vi "test_read-nmea-data2.vi"() -> ()   [LabVIEW 2019]
uses:
  <vilib>/Utility/file.llb/Write Delimited Spreadsheet (string).vi
panel:
  out "Array 2":string[](array[string])
  out "Numeric":i32=9674
  out "Array":string[](array[string])
  out "before substring":string
  in  "text":string="15:08:57.26\tF9P\t$GNRMC,060859.00,A,3723.60792,N,12656.91690,E,0.042,,250720,,,A,V*1C\n\t\n15:08:57.28\tF9P\t$GNVTG,,T,,M,0.042,N,0.078,K,A*34\n\t\n15:08:57.30\tF9P\t$GNGGA,060859.00,3723.60792,N,12656.91690,E,1,12,0.63,59.1,M,18.5,M,,*79\n\t\n15:08:57.32\tF9P\t$GNGSA,A,3,12,06,19,05,17,09,04,02,,,,,1.16,0.63,0.97,1*0D\n\t\n15:08:57.34\tF9P\t$GNGSA,A,3,70,85,71,84,,,,,,,,,1.16,0.63,0.97,2*0F\n\t\n15:08:57.36\tF9P\t$GNGSA,A,3,36,19,11,04,09,12,,,,,,,1.16,0.63,0.97,3*0D\n\t\n15:08:57.38\tF9P\t$GNGSA,A,3,14,11,33,,,,,,,,,,1.16,0.63,0.97,4*0C\n\t\n15:08:57.40\tF9P\t$GPGSV,3,1,09,02,53,317,32,04,19,045,33,05,36,246,36,06,65,044,35,1*64\n\t\n15:08:57.42\tF9P\t$GPGSV,3,2,09,09,45,076,33,12,24,278,37,17,35,153,31,19,54,156,27,1*62\n\t\n15:08:57.44\tF9P\t$GPGSV,3,3,09,25,12,308,17,1*54\n\t\n15:08:57.46\tF9P\t$GPGSV,3,1,09,02,53,317,,04,19,045,25,05,36,246,25,06,65,044,23,6*60\n\t\n15:08:57.48\tF9P\t$GPGSV,3,2,09,09,45,076,27,12,24,278,13,17,35,153,14,19,54,156,,6*64\n\t\n15:08:57.50\tF9P\t$GPGSV,3,3,09,25,12,308,,6*55\n\t\n15:08:57.52\tF9P\t$GLGSV,2,1,08,69,13,031,,70,73,042,31,71,50,204,30,72,03,209,,1*70\n\t\n15:08:57.54\tF9P\t$GLGSV,2,2,08,77,01,327,,84,21,121,18,85,70,063,38,86,35,329,,1*77\n\t\n15:08:57.56\tF9P\t$GLGSV,2,1,08,69,13,031,,70,73,042,,71,50,204,27,72,03,209,,3*76\n\t\n15:08:57.58\tF9P\t$GLGSV,2,2,08,77,01,327,,84,21,121,22,85,70,063,30,86,35,329,,3*74\n\t\n15:08:57.60\tF9P\t$GAGSV,2,1,08,02,09,298,09,04,65,120,29,09,30,193,23,11,70,356,33,7*71\n\t\n15:08:57.62\tF9P\t$GAGSV,2,2,08,12,41,101,23,19,27,046,24,25,10,250,,36,25,307,18,7*7B\n\t\n15:08:57.64\tF9P\t$GAGSV,2,1,08,02,09,298,,04,65,120,31,09,30,193,,11,70,356,20,2*77\n\t\n15:08:57.66\tF9P\t$GAGSV,2,2,08,12,41,101,25,19,27,046,18,25,10,250,,36,25,307,25,2*79\n\t\n15:08:57.68\tF9P\t$GBGSV,1,1,03,11,51,130,31,14,86,148,35,33,59,218,41,1*43\n\t\n15:08:57.70\tF9P\t$GBGSV,2,1,05,08,,,29,10,,,10,11,51,130,36,14,86,148,29,3*7F\n\t\n15:08:57.72\tF9P\t$GBGSV,2,2,05,33,59,218,,3*46\n\t\n15:08:57.74\tF9P\t$GNGLL,3723.60792,N,12656.91690,E,060859.00,A,A*7B\n\t\n15:08:57.76\tF9P\t\t\n15:08:57.78\tF9P\t\t\n15:08:57.80\tF9P\t\t\n15:08:57.82\tF9P\t\t\n15:08:57.84\tF9P\t\t\n15:08:57.86\tF9P\t\t\n15:08:57.88\tF9P\t\t\n15:08:57.90\tF9P\t\t\n15:08:57.92\tF9P\t\t\n15:08:57.94\tF9P\t\t\n15:08:57.96\tF9P\t\t\n15:08:57.98\tF9P\t\t\n15:08:58.00\tF9P\t\t\n15:08:58.02\tF9P\t\t\n15:08:58.04\tF9P\t\t\n15:08:58.06\tF9P\t\t\n15:08:58.08\tF9P\t\t\n15:08:58.10\tF9P\t\t\n15:08:58.12\tF9P\t\t\n15:08:58.14\tF9P\t\t\n15:08:58.16\tF9P\t\t\n15:08:58.18\tF9P\t\t\n15:08:58.20\tF9P\t\t\n15:08:58.22\tF9P\t\t\n15:08:58.24\tF9P\t\t\n15:08:58.26\tF9P\t$GNRMC,060900.00,A,3723.60793,N,12656.91687,E,0.035,,250720,,,A,V*16\n\t\n15:08:58.28\tF9P\t$GNVTG,,T,,M,0.035,N,0.066,K,A*3B\n\t\n15:08:58.30\tF9P\t$GNGGA,060900.00,3723.60793,N,12656.91687,E,1,12,0.68,59.2,M,18.5,M,,*7B\n\t\n15:08:58.32\tF9P\t$GNGSA,A,3,12,06,19,05,17,09,04,02,,,,,1.22,0.68,1.01,1*0F\n\t\n15:08:58.34\tF9P\t$GNGSA,A,3,70,85,71,84,,,,,,,,,1.22,0.68,1.01,2*0D\n\t\n15:08:58.36\tF9P\t$GNGSA,A,3,36,19,11,04,09,12,,,,,,,1.22,0.68,1.01,3*0F\n\t\n15:08:58.38\tF9P\t$GNGSA,A,3,14,11,33,,,,,,,,,,1.22,0.68,1.01,4*0E\n\t\n15:08:58.40\tF9P\t$GPGSV,3,1,09,02,53,317,26,04,19,045,33,05,36,246,33,06,65,044,30,1*61\n\t\n15:08:58.42\tF9P\t$GPGSV,3,2,09,09,45,076,29,12,24,278,38,17,35,153,31,19,54,156,25,1*64\n\t\n15:08:58.44\tF9P\t$GPGSV,3,3,09,25,12,308,17,1*54\n\t\n15:08:58.46\tF9P\t$GPGSV,3,1,09,02,53,317,,04,19,045,26,05,36,246,25,06,65,044,24,6*64\n\t\n15:08:58.48\tF9P\t$GPGSV,3,2,09,09,45,076,27,12,24,278,14,17,35,153,14,19,54,156,,6*63\n\t\n15:08:58.50\tF9P\t$GPGSV,3,3,09,25,12,308,,6*55\n\t\n15:08:58.52\tF9P\t$GLGSV,2,1,08,69,13,031,,70,73,042,29,71,50,204,31,72,03,209,,1*78\n\t\n15:08:58.54\tF9P\t$GLGSV,2,2,08,77,01,327,,84,21,121,16,85,70,063,34,86,35,329,,1*75\n\t\n15:08:58.56\tF9P\t$GLGSV,2,1,08,69,13,031,,70,73,042,,71,50,204,26,72,03,209,,3*77\n\t\n15:08:58.58\tF9P\t$GLGSV,2,2,08,77,01,327,,84,21,121,22,85,70,063,29,86,35,329,,3*7C\n\t\n15:08:58.60\tF9P\t$GAGSV,2,1,08,02,09,298,06,04,65,120,29,09,30,193,23,11,70,356,31,7*7C\n\t\n15:08:58.62\tF9P\t$GAGSV,2,2,08,12,41,101,25,19,27,046,22,25,10,250,,36,25,307,17,7*74\n\t\n15:08:58.64\tF9P\t$GAGSV,2,1,08,02,09,298,,04,65,120,30,09,30,193,,11,70,356,19,2*7C\n\t\n15:08:58.66\tF9P\t$GAGSV,2,2,08,12,41,101,24,19,27,046,20,25,10,250,,36,25,307,23,2*75\n\t\n15:08:58.68\tF9P\t$GBGSV,1,1,03,11,51,130,31,14,86,148,32,33,59,218,39,1*4B\n\t\n15:08:58.70\tF9P\t$GBGSV,2,1,05,08,,,28,10,,,09,11,51,130,36,14,86,148,28,3*77\n\t\n15:08:58.72\tF9P\t$GBGSV,2,2,05,33,59,218,,3*46\n\t\n15:08:58.74\tF9P\t$GNGLL,3723.60793,N,12656.91687,E,060900.00,A,A*71\n\t\n15:08:58.76\tF9P\t\t\n15:08:58.78\tF9P\t\t\n15:08:58.80\tF9P\t\t\n15:08:58.82\tF9P\t\t\n15:08:58.84\tF9P\t\t\n15:08:58.86\tF9P\t\t\n15:08:58.88\tF9P\t\t\n15:08:58.90\tF9P\t\t\n15:08:58.92\tF9P\t\t\n15:08:58.94\tF9P\t\t\n15:08:58.96\tF9P\t\t\n15:08:58.98\tF9P\t\t\n15:08:59.00\tF9P\t\t\n15:08:59.02\tF9P\t\t\n15:08:59.04\tF9P\t\t\n15:08:59.06\tF9P\t\t\n15:08:59.08\tF9P\t\t\n15:08:59.10\tF9P\t\t\n15:08:59.12\tF9P\t\t\n15:08:59.14\tF9P\t\t\n15:08:59.16\tF9P\t\t\n15:08:59.18\tF9P\t\t\n15:08:59.20\tF9P\t\t\n15:08:59.22\tF9P\t\t\n15:08:59.24\tF9P\t\t\n15:08:59.26\tF9P\t$GNRMC,060901.00,A,3723.60794,N,12656.91683,E,0.044,,250720,,,A,V*12\n\t\n15:08:59.28\tF9P\t$GNVTG,,T,,M,0.044,N,0.082,K,A*37\n\t\n15:08:59.30\tF9P\t$GNGGA,060901.00,3723.60794,N,12656.91683,E,1,12,0.68,59.2,M,18.5,M,,*79\n\t\n15:08:59.32\tF9P\t$GNGSA,A,3,12,06,19,05,17,09,04,02,,,,,1.22,0.68,1.01,1*0F\n\t\n15:08:59.34\tF9P\t$GNGSA,A,3,70,85,71,84,,,,,,,,,1.22,0.68,1.01,2*0D\n\t\n15:08:59.36\tF9P\t$GNGSA,A,3,36,19,11,04,09,12,,,,,,,1.22,0.68,1.01,3*0F\n\t\n15:08:59.38\tF9P\t$GNGSA,A,3,14,11,33,,,,,,,,,,1.22,0.68,1.01,4*0E\n\t\n15:08:59.40\tF9P\t$GPGSV,3,1,09,02,53,317,28,04,19,045,33,05,36,246,34,06,65,044,34,1*6C\n\t\n15:08:59.42\tF9P\t$GPGSV,3,2,09,09,45,076,31,12,24,278,38,17,35,153,30,19,54,156,26,1*6F\n\t\n15:08:59.44\tF9P\t$GPGSV,3,3,09,25,12,308,18,1*5B\n\t\n15:08:59.46\tF9P\t$GPGSV,3,1,09,02,53,317,,04,19,045,26,05,36,246,25,06,65,044,25,6*65\n\t\n15:08:59.49\tF9P\t$GPGSV,3,2,09,09,45,076,27,12,24,278,13,17,35,153,16,19,54,156,,6*66\n\t\n15:08:59.51\tF9P\t$GPGSV,3,3,09,25,12,308,,6*55\n\t\n15:08:59.53\tF9P\t$GLGSV,2,1,08,69,13,031,,70,73,042,29,71,50,204,22,72,03,209,,1*7A\n\t\n15:08:59.55\tF9P\t$GLGSV,2,2,08,77,01,327,,84,21,121,13,85,70,063,33,86,35,329,,1*77\n\t\n15:08:59.57\tF9P\t$GLGSV,2,1,08,69,13,031,,70,73,042,,71,50,204,25,72,03,209,,3*74\n\t\n15:08:59.59\tF9P\t$GLGSV,2,2,08,77,01,327,,84,21,121,23,85,70,063,27,86,35,329,,3*73\n\t\n15:08:59.61\tF9P\t$GAGSV,2,1,08,02,09,298,09,04,65,120,34,09,30,193,25,11,70,356,31,7*79\n\t\n15:08:59.63\tF9P\t$GAGSV,2,2,08,12,41,101,22,19,27,046,21,25,10,250,,36,25,307,16,7*71\n\t\n15:08:59.65\tF9P\t$GAGSV,2,1,08,02,09,298,,04,65,120,30,09,30,193,,11,70,356,20,2*76\n\t\n15:08:59.67\tF9P\t$GAGSV,2,2,08,12,41,101,24,19,27,046,21,25,10,250,,36,25,307,23,2*74\n\t\n15:08:59.69\tF9P\t$GBGSV,1,1,03,11,51,130,32,14,86,148,34,33,59,218,40,1*40\n\t\n15:08:59.71\tF9P\t$GBGSV,2,1,05,08,,,27,10,,,08,11,51,130,36,14,86,148,26,3*77\n\t\n15:08:59.73\tF9P\t$GBGSV,2,2,05,33,59,218,,3*46\n\t\n15:08:59.75\tF9P\t$GNGLL,3723.60794,N,12656.91683,E,060901.00,A,A*73\n\t\n15:08:59.77\tF9P\t\t\n15:08:59.79\tF9P\t\t\n15:08:59.81\tF9P\t\t\n15:08:59.83\tF9P\t\t\n15:08:59.85\tF9P\t\t\n15:08:59.87\tF9P\t\t\n15:08:59.89\tF9P\t\t\n15:08:59.91\tF9P\t\t\n15:08:59.93\tF9P\t\t\n15:08:59.95\tF9P\t\t\n15:08:59.97\tF9P\t\t\n15:08:59.99\tF9P\t\t\n15:09:00.01\tF9P\t\t\n15:09:00.03\tF9P\t\t\n15:09:00.05\tF9P\t\t\n15:09:00.07\tF9P\t\t\n15:09:00.09\tF9P\t\t\n15:09:00.11\tF9P\t\t\n15:09:00.13\tF9P\t\t\n15:09:00.15\tF9P\t\t\n15:09:00.17\tF9P\t\t\n15:09:00.19\tF9P\t\t\n15:09:00.21\tF9P\t\t\n15:09:00.23\tF9P\t\t\n15:09:00.25\tF9P\t$GNRMC,060902.00,A,3723.60796,N,12656.91700,E,0.733,,250720,,,A,V*1E\n\t\n15:09:00.27\tF9P\t$GNVTG,,T,,M,0.733,N,1.358,K,A*35\n\t\n15:09:00.29\tF9P\t$GNGGA,060902.00,3723.60796,N,12656.91700,E,1,12,0.72,59.0,M,18.5,M,,*7B\n\t\n15:09:00.31\tF9P\t$GNGSA,A,3,12,06,19,05,17,09,04,02,,,,,1.25,0.72,1.02,1*00\n\t\n15:09:00.33\tF9P\t$GNGSA,A,3,70,85,71,84,,,,,,,,,1.25,0.72,1.02,2*02\n\t\n15:09:00.35\tF9P\t$GNGSA,A,3,36,19,11,04,09,12,,,,,,,1.25,0.72,1.02,3*00\n\t\n15:09:00.37\tF9P\t$GNGSA,A,3,14,11,33,,,,,,,,,,1.25,0.72,1.02,4*01\n\t\n15:09:00.39\tF9P\t$GPGSV,3,1,09,02,54,318,27,04,19,045,28,05,36,246,35,06,65,044,33,1*67\n\t\n15:09:00.41\tF9P\t$GPGSV,3,2,09,09,45,076,23,12,24,278,30,17,35,153,29,19,54,156,31,1*6A\n\t\n15:09:00.43\tF9P\t$GPGSV,3,3,09,25,12,308,17,1*54\n\t\n15:09:00.45\tF9P\t$GPGSV,3,1,09,02,54,318,,04,19,045,25,05,36,246,24,06,65,044,23,6*69\n\t\n15:09:00.47\tF9P\t$GPGSV,3,2,09,09,45,076,26,12,24,278,21,17,35,153,15,19,54,156,,6*65\n\t\n15:09:00.49\tF9P\t$GPGSV,3,3,09,25,12,308,,6*55\n\t\n15:09:00.51\tF9P\t$GLGSV,2,1,08,69,13,031,,70,73,042,29,71,50,204,29,72,03,209,,1*71\n\t\n15:09:00.53\tF9P\t$GLGSV,2,2,08,77,01,327,,84,21,121,18,85,70,063,33,86,35,329,,1*7C\n\t\n15:09:00.55\tF9P\t$GLGSV,2,1,08,69,13,031,,70,73,042,,71,50,204,25,72,03,209,,3*74\n\t\n15:09:00.57\tF9P\t$GLGSV,2,2,08,77,01,327,,84,21,121,22,85,70,063,26,86,35,329,,3*73\n\t\n15:09:00.59\tF9P\t$GAGSV,2,1,08,02,09,298,12,04,65,120,30,09,30,193,31,11,70,356,27,7*75\n\t\n15:09:00.61\tF9P\t$GAGSV,2,2,08,12,41,101,22,19,27,046,22,25,10,250,,36,25,307,19,7*7D\n\t\n15:09:00.63\tF9P\t$GAGSV,2,1,08,02,09,298,,04,65,120,23,09,30,193,,11,70,356,24,2*70\n\t\n15:09:00.65\tF9P\t$GAGSV,2,2,08,12,41,101,23,19,27,046,21,25,10,250,,36,25,307,21,2*71\n\t\n15:09:00.67\tF9P\t$GBGSV,1,1,03,11,51,130,24,14,86,148,28,33,59,218,34,1*49\n\t\n15:09:00.69\tF9P\t$GBGSV,2,1,05,08,,,26,10,,,08,11,51,130,22,14,86,148,26,3*73\n\t\n15:09:00.71\tF9P\t$GBGSV,2,2,05,33,59,218,,3*46\n\t\n15:09:00.73\tF9P\t$GNGLL,3723.60796,N,12656.91700,E,060902.00,A,A*78\n\t\n15:09:00.75\tF9P\t\t\n15:09:00.77\tF9P\t\t\n15:09:00.79\tF9P\t\t\n15:09:00.81\tF9P\t\t\n15:09:00.83\tF9P\t\t\n15:09:00.85\tF9P\t\t\n15:09:00.87\tF9P\t\t\n15:09:00.89\tF9P\t\t\n15:09:00.91\tF9P\t\t\n15:09:00.93\tF9P\t\t\n15:09:00.95\tF9P\t\t\n15:09:00.97\tF9P\t\t\n15:09:00.99\tF9P\t\t\n15:09:01.01\tF9P\t\t\n15:09:01.03\tF9P\t\t\n15:09:01.05\tF9P\t\t\n15:09:01.07\tF9P\t\t\n15:09:01.09\tF9P\t\t\n15:09:01.11\tF9P\t\t\n15:09:01.13\tF9P\t\t\n15:09:01.15\tF9P\t\t\n15:09:01.17\tF9P\t\t\n15:09:01.19\tF9P\t\t\n15:09:01.21\tF9P\t\t\n15:09:01.23\tF9P\t\t\n15:09:01.25\tF9P\t$GNRMC,060903.00,A,3723.60797,N,12656.91717,E,0.183,,250720,,,A,V*15\n\t\n15:09:01.27\tF9P\t$GNVTG,,T,,M,0.183,N,0.340,K,A*30\n\t\n15:09:01.29\tF9P\t$GNGGA,060903.00,3723.60797,N,12656.91717,E,1,12,0.68,59.0,M,18.5,M,,*76\n\t\n15:09:01.31\tF9P\t$GNGSA,A,3,12,06,19,05,17,09,04,02,,,,,1.22,0.68,1.01,1*0F\n\t\n15:09:01.33\tF9P\t$GNGSA,A,3,70,85,71,84,,,,,,,,,1.22,0.68,1.01,2*0D\n\t\n15:09:01.35\tF9P\t$GNGSA,A,3,36,19,11,04,09,12,,,,,,,1.22,0.68,1.01,3*0F\n\t\n15:09:01.37\tF9P\t$GNGSA,A,3,14,11,33,,,,,,,,,,1.22,0.68,1.01,4*0E\n\t\n15:09:01.39\tF9P\t$GPGSV,3,1,09,02,54,318,31,04,19,045,28,05,36,246,29,06,65,044,33,1*6D\n\t\n15:09:01.41\tF9P\t$GPGSV,3,2,09,09,45,076,34,12,24,278,33,17,35,153,28,19,54,156,26,1*68\n\t\n15:09:01.43\tF9P\t$GPGSV,3,3,09,25,12,308,16,1*55\n\t\n15:09:01.45\tF9P\t$GPGSV,3,1,09,02,54,318,,04,19,045,22,05,36,246,20,06,65,044,21,6*68\n\t\n15:09:01.47\tF9P\t$GPGSV,3,2,09,09,45,076,24,12,24,278,22,17,35,153,13,19,54,156,,6*62\n\t\n15:09:01.49\tF9P\t$GPGSV,3,3,09,25,12,308,,6*55\n\t\n15:09:01.51\tF9P\t$GLGSV,2,1,08,69,13,031,,70,73,042,20,71,50,204,20,72,03,209,,1*71\n\t\n15:09:01.53\tF9P\t$GLGSV,2,2,08,77,01,327,,84,21,121,12,85,70,063,29,86,35,329,,1*7D\n\t\n15:09:01.55\tF9P\t$GLGSV,2,1,08,69,13,031,,70,73,042,,71,50,204,22,72,03,209,,3*73\n\t\n15:09:01.57\tF9P\t$GLGSV,2,2,08,77,01,327,,84,21,121,23,85,70,063,25,86,35,329,,3*71\n\t\n15:09:01.59\tF9P\t$GAGSV,2,1,08,02,09,298,12,04,65,120,31,09,30,193,24,11,70,356,35,7*73\n\t\n15:09:01.61\tF9P\t$GAGSV,2,2,08,12,41,101,21,19,27,046,31,25,10,250,,36,25,307,18,7*7D\n\t\n15:09:01.63\tF9P\t$GAGSV,2,1,08,02,09,298,,04,65,120,29,09,30,193,,11,70,356,24,2*7A\n\t\n15:09:01.65\tF9P\t$GAGSV,2,2,08,12,41,101,24,19,27,046,21,25,10,250,,36,25,307,19,2*7D\n\t\n15:09:01.67\tF9P\t$GBGSV,1,1,03,11,51,130,18,14,86,148,24,33,59,218,25,1*4A\n\t\n15:09:01.69\tF9P\t$GBGSV,2,1,05,08,,,32,10,,,08,11,51,130,20,14,86,148,26,3*74\n\t\n15:09:01.71\tF9P\t$GBGSV,2,2,05,33,59,218,,3*46\n\t\n15:09:01.73\tF9P\t$GNGLL,3723.60797,N,12656.91717,E,060903.00,A,A*7E\n\t\n15:09:01.75\tF9P\t\t\n15:09:01.77\tF9P\t\t\n15:09:01.79\tF9P\t\t\n15:09:01.81\tF9P\t\t\n15:09:01.83\tF9P\t\t\n15:09:01.85\tF9P\t\t\n15:09:01.87\tF9P\t\t\n15:09:01.89\tF9P\t\t\n15:09:01.91\tF9P\t\t\n15:09:01.93\tF9P\t\t\n15:09:01.95\tF9P\t\t\n15:09:01.97\tF9P\t\t\n15:09:01.99\tF9P\t\t\n15:09:02.01\tF9P\t\t\n15:09:02.03\tF9P\t\t\n15:09:02.05\tF9P\t\t\n15:09:02.07\tF9P\t\t\n15:09:02.09\tF9P\t\t\n15:09:02.11\tF9P\t\t\n15:09:02.13\tF9P\t\t\n15:09:02.15\tF9P\t\t\n15:09:02.17\tF9P\t\t\n15:09:02.19\tF9P\t\t\n15:09:02.21\tF9P\t\t\n15:09:02.23\tF9P\t\t\n15:09:02.25\tF9P\t$GNRMC,060904.00,A,3723.60804,N,12656.91741,E,0.193,,250720,,,A,V*15\n\t\n15:09:02.27\tF9P\t$GNVTG,,T,,M,0.193,N,0.358,K,A*38\n\t\n15:09:02.29\tF9P\t$GNGGA,060904.00,3723.60804,N,12656.91741,E,1,12,0.72,58.8,M,18.5,M,,*75\n\t\n15:09:02.31\tF9P\t$GNGSA,A,3,12,06,19,05,17,09,04,02,,,,,1.25,0.72,1.02,1*00\n\t\n15:09:02.33\tF9P\t$GNGSA,A,3,70,85,71,84,,,,,,,,,1.25,0.72,1.02,2*02\n\t\n15:09:02.35\tF9P\t$GNGSA,A,3,36,19,11,04,09,12,,,,,,,1.25,0.72,1.02,3*00\n\t\n15:09:02.37\tF9P\t$GNGSA,A,3,14,11,33,,,,,,,,,,1.25,0.72,1.02,4*01\n\t\n15:09:02.39\tF9P\t$GPGSV,3,1,09,02,54,318,25,04,19,044,29,05,36,246,29,06,65,044,36,1*6D\n\t\n15:09:02.41\tF9P\t$GPGSV,3,2,09,09,45,076,39,12,24,278,30,17,35,153,16,19,54,156,27,1*6A\n\t\n15:09:02.43\tF9P\t$GPGSV,3,3,09,25,12,308,14,1*57\n\t\n15:09:02.45\tF9P\t$GPGSV,3,1,09,02,54,318,,04,19,044,17,05,36,246,15,06,65,044,22,6*6A\n\t\n15:09:02.47\tF9P\t$GPGSV,3,2,09,09,45,076,20,12,24,278,22,17,35,153,10,19,54,156,,6*65\n\t\n15:09:02.49\tF9P\t$GPGSV,3,3,09,25,12,308,,6*55\n\t\n15:09:02.51\tF9P\t$GLGSV,2,1,08,69,13,031,,70,73,042,20,71,50,204,20,72,03,209,,1*71\n\t\n15:09:02.53\tF9P\t$GLGSV,2,2,08,77,01,327,,84,21,121,12,85,70,063,29,86,35,329,,1*7D\n\t\n15:09:02.55\tF9P\t$GLGSV,2,1,08,69,13,031,,70,73,042,,71,50,204,20,72,03,209,,3*71\n\t\n15:09:02.57\tF9P\t$GLGSV,2,2,08,77,01,327,,84,21,121,23,85,70,063,25,86,35,329,,3*71\n\t\n15:09:02.59\tF9P\t$GAGSV,2,1,08,02,09,298,08,04,65,120,35,09,30,193,25,11,70,356,32,7*7A\n\t\n15:09:02.61\tF9P\t$GAGSV,2,2,08,12,41,101,21,19,27,046,33,25,10,250,,36,25,307,17,7*70\n\t\n15:09:02.63\tF9P\t$GAGSV,2,1,08,02,09,298,,04,65,120,23,09,30,193,,11,70,356,23,2*77\n\t\n15:09:02.65\tF9P\t$GAGSV,2,2,08,12,41,101,23,19,27,046,20,25,10,250,,36,25,307,15,2*77\n\t\n15:09:02.67\tF9P\t$GBGSV,1,1,03,11,51,130,25,14,86,148,31,33,59,218,25,1*40\n\t\n15:09:02.69\tF9P\t$GBGSV,2,1,05,08,,,35,10,,,08,11,51,130,21,14,86,148,25,3*71\n\t\n15:09:02.71\tF9P\t$GBGSV,2,2,05,33,59,218,,3*46\n\t\n15:09:02.73\tF9P\t$GNGLL,3723.60804,N,12656.91741,E,060904.00,A,A*7F\n\t\n15:09:02.75\tF9P\t\t\n15:09:02.77\tF9P\t\t\n15:09:02.79\tF9P\t\t\n15:09:02.81\tF9P\t\t\n15:09:02.83\tF9P\t\t\n15:09:02.85\tF9P\t\t\n15:09:02.87\tF9P\t\t\n15:09:02.89\tF9P\t\t\n15:09:02.91\tF9P\t\t\n15:09:02.93\tF9P\t\t\n15:09:02.95\tF9P\t\t\n15:09:02.97\tF9P\t\t\n15:09:02.99\tF9P\t\t\n15:09:03.01\tF9P\t\t\n15:09:03.03\tF9P\t\t\n15:09:03.05\tF9P\t\t\n15:09:03.07\tF9P\t\t\n15:09:03.09\tF9P\t\t\n15:09:03.11\tF9P\t\t\n15:09:03.13\tF9P\t\t\n15:09:03.15\tF9P\t\t\n15:09:03.17\tF9P\t\t\n15:09:03.19\tF9P\t\t\n15:09:03.21\tF9P\t\t\n15:09:03.23\tF9P\t\t\n15:09:03.25\tF9P\t$GNRMC,060905.00,A,3723.60816,N,12656.91764,E,0.775,,250720,,,A,V*1E\n\t\n15:09:03.27\tF9P\t$GNVTG,,T,,M,0.775,N,1.436,K,A*38\n\t\n15:09:03.29\tF9P\t$GNGGA,060905.00,3723.60816,N,12656.91764,E,1,12,0.68,58.8,M,18.5,M,,*7B\n\t\n15:09:03.31\tF9P\t$GNGSA,A,3,12,06,19,05,17,09,04,02,,,,,1.22,0.68,1.01,1*0F\n\t\n15:09:03.33\tF9P\t$GNGSA,A,3,70,85,71,84,,,,,,,,,1.22,0.68,1.01,2*0D\n\t\n15:09:03.35\tF9P\t$GNGSA,A,3,36,19,11,04,09,12,,,,,,,1.22,0.68,1.01,3*0F\n\t\n15:09:03.37\tF9P\t$GNGSA,A,3,14,11,33,,,,,,,,,,1.22,0.68,1.01,4*0E\n\t\n15:09:03.39\tF9P\t$GPGSV,3,1,09,02,54,318,27,04,19,044,33,05,36,246,26,06,65,044,37,1*6A\n\t\n15:09:03.41\tF9P\t$GPGSV,3,2,09,09,45,076,27,12,24,278,28,17,35,153,19,19,54,156,27,1*63\n\t\n15:09:03.43\tF9P\t$GPGSV,3,3,09,25,12,308,,1*52\n\t\n15:09:03.45\tF9P\t$GPGSV,3,1,09,02,54,318,,04,19,044,18,05,36,246,14,06,65,044,30,6*67\n\t\n15:09:03.47\tF9P\t$GPGSV,3,2,09,09,45,076,27,12,24,278,22,17,35,153,,19,54,156,,6*63\n\t\n15:09:03.49\tF9P\t$GPGSV,3,3,09,25,12,308,,6*55\n\t\n15:09:03.51\tF9P\t$GLGSV,2,1,08,69,13,031,,70,73,042,22,71,50,204,30,72,03,209,,1*72\n\t\n15:09:03.53\tF9P\t$GLGSV,2,2,08,77,01,327,,84,21,121,06,85,70,063,33,86,35,329,,1*73\n\t\n15:09:03.55\tF9P\t$GLGSV,2,1,08,69,13,031,,70,73,042,,71,50,204,19,72,03,209,,3*7B\n\t\n15:09:03.57\tF9P\t$GLGSV,2,2,08,77,01,327,,84,21,121,22,85,70,063,25,86,35,329,,3*70\n\t\n15:09:03.59\tF9P\t$GAGSV,2,1,08,02,09,298,11,04,65,120,27,09,30,193,24,11,70,356,28,7*7B\n\t\n15:09:03.61\tF9P\t$GAGSV,2,2,08,12,41,101,22,19,27,046,27,25,10,250,,36,25,307,17,7*76\n\t\n15:09:03.63\tF9P\t$GAGSV,2,1,08,02,09,298,,04,65,120,29,09,30,193,,11,70,356,31,2*7E\n\t\n15:09:03.65\tF9P\t$GAGSV,2,2,08,12,41,101,22,19,27,046,20,25,10,250,,36,25,307,13,2*70\n\t\n15:09:03.67\tF9P\t$GBGSV,1,1,03,11,51,130,28,14,86,148,27,33,59,218,27,1*48\n\t\n15:09:03.69\tF9P\t$GBGSV,2,1,05,08,,,28,10,,,08,11,51,130,30,14,86,148,35,3*7C\n\t\n15:09:03.71\tF9P\t$GBGSV,2,2,05,33,59,218,,3*46\n\t\n15:09:03.73\tF9P\t$GNGLL,3723.60816,N,12656.91764,E,060905.00,A,A*7A\n\t\n15:09:03.75\tF9P\t\t\n15:09:03.77\tF9P\t\t\n15:09:03.79\tF9P\t\t\n15:09:03.81\tF9P\t\t\n15:09:03.83\tF9P\t\t\n15:09:03.85\tF9P\t\t\n15:09:03.87\tF9P\t\t\n15:09:03.89\tF9P\t\t\n15:09:03.91\tF9P\t\t\n15:09:03.93\tF9P\t\t\n15:09:03.95\tF9P\t\t\n15:09:03.97\tF9P\t\t\n15:09:03.99\tF9P\t\t\n15:09:04.01\tF9P\t\t\n15:09:04.03\tF9P\t\t\n15:09:04.05\tF9P\t\t\n15:09:04.07\tF9P\t\t\n15:09:04.09\tF9P\t\t\n15:09:04.11\tF9P\t\t\n15:09:04.13\tF9P\t\t\n15:09:04.15\tF9P\t\t\n15:09:04.17\tF9P\t\t\n15:09:04.19\tF9P\t\t\n15:09:04.21\tF9P\t\t\n15:09:04.23\tF9P\t\t\n15:09:04.25\tF9P\t$GNRMC,060906.00,A,3723.60830,N,12656.91746,E,1.017,354.28,250720,,,A,V*0D\n\t\n15:09:04.27\tF9P\t$GNVTG,354.28,T,,M,1.017,N,1.884,K,A*29\n\t\n15:09:04.29\tF9P\t$GNGGA,060906.00,3723.60830,N,12656.91746,E,1,12,0.72,59.0,M,18.5,M,,*7E\n\t\n15:09:04.31\tF9P\t$GNGSA,A,3,12,06,19,05,17,09,04,02,,,,,1.25,0.72,1.02,1*00\n\t\n15:09:04.33\tF9P\t$GNGSA,A,3,70,85,71,84,,,,,,,,,1.25,0.72,1.02,2*02\n\t\n15:09:04.35\tF9P\t$GNGSA,A,3,36,19,11,04,09,12,,,,,,,1.25,0.72,1.02,3*00\n\t\n15:09:04.37\tF9P\t$GNGSA,A,3,14,11,33,,,,,,,,,,1.25,0.72,1.02,4*01\n\t\n15:09:04.39\tF9P\t$GPGSV,3,1,09,02,54,318,26,04,19,044,28,05,36,246,25,06,65,046,27,1*61\n\t\n15:09:04.41\tF9P\t$GPGSV,3,2,09,09,45,076,27,12,24,278,28,17,35,153,22,19,54,156,26,1*6A\n\t\n15:09:04.43\tF9P\t$GPGSV,3,3,09,25,12,308,,1*52\n\t\n15:09:04.45\tF9P\t$GPGSV,3,1,09,02,54,318,,04,19,044,21,05,36,246,16,06,65,046,21,6*6D\n\t\n15:09:04.48\tF9P\t$GPGSV,3,2,09,09,45,076,21,12,24,278,21,17,35,153,,19,54,156,,6*66\n\t\n15:09:04.50\tF9P\t$GPGSV,3,3,09,25,12,308,,6*55\n\t\n15:09:04.52\tF9P\t$GLGSV,2,1,08,69,13,031,,70,73,042,23,71,50,204,33,72,03,209,,1*70\n\t\n15:09:04.54\tF9P\t$GLGSV,2,2,08,77,01,327,,84,21,121,10,85,70,063,23,86,35,329,,1*75\n\t\n15:09:04.56\tF9P\t$GLGSV,2,1,08,69,13,031,,70,73,042,,71,50,204,20,72,03,209,,3*71\n\t\n15:09:04.58\tF9P\t$GLGSV,2,2,08,77,01,327,,84,21,121,19,85,70,063,23,86,35,329,,3*7E\n\t\n15:09:04.60\tF9P\t$GAGSV,2,1,08,02,09,298,11,04,65,120,25,09,30,193,24,11,70,356,26,7*77\n\t\n15:09:04.62\tF9P\t$GAGSV,2,2,08,12,41,101,23,19,27,046,26,25,10,250,,36,25,307,17,7*76\n\t\n15:09:04.64\tF9P\t$GAGSV,2,1,08,02,09,298,,04,65,120,29,09,30,193,,11,70,356,27,2*79\n\t\n15:09:04.66\tF9P\t$GAGSV,2,2,08,12,41,101,21,19,27,046,20,25,10,250,,36,25,307,12,2*72\n\t\n15:09:04.68\tF9P\t$GBGSV,1,1,03,11,51,130,27,14
